vi "Remove Unused Connections.vi"(11 "TCP Slave in":refnum<class "TCP Server.lvclass">) -> (0 "error out":errorcluster)   [LabVIEW 2021, in "WebSockets.lvlib" / "TCP Server.lvclass"]
uses:
  TCP Server.lvclass
  TCP Server.lvclass/TCP Server.ctl
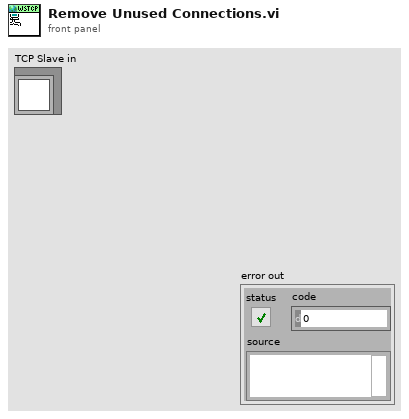
[diagram p1: front panel]
types:
  T1 = typedef "WebSockets.lvlib/TCP Server.lvclass/Connection Counter.ctl" = cluster{"Currently Connected":u32, "Connection Records":refnum<data-value>[]}
  T2 = typedef "WebSockets.lvlib/TCP Server.lvclass/Connection.ctl" = cluster{"Connected?":bool, "IP address":string, "connection error":errorcluster}
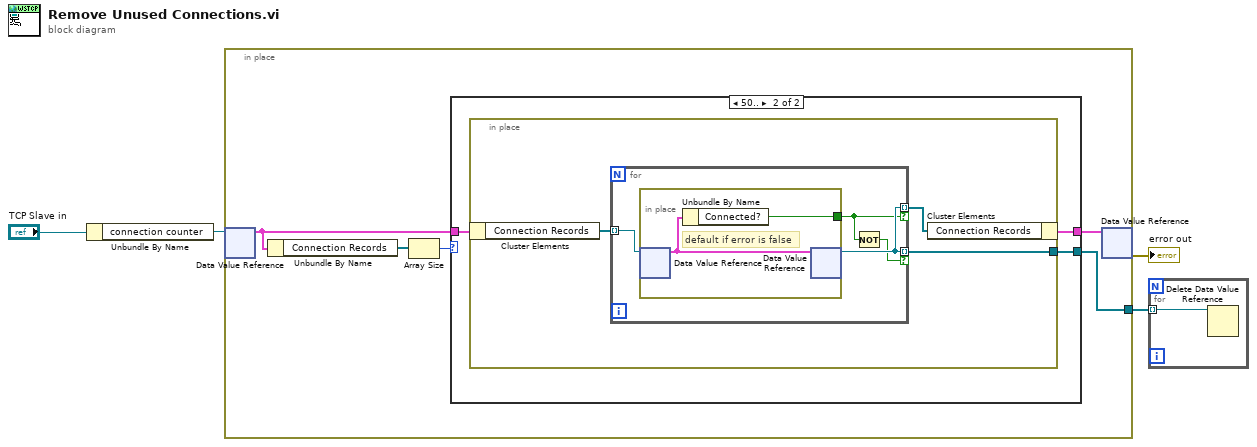
[diagram p0: block diagram]
diagram:
  n1 = Unbundle By Name("TCP Slave in") -> ("connection counter"=w2:refnum<data-value>)
  n2 = in-place {
    in-place-border: [w5] -> w1
    n3 = in-place-dvr #1(w2) -> (w6:T1)  [unwired: 1 out]
    n4 = Unbundle By Name(w6) -> ("Connection Records"=w8:refnum<data-value>[])
    n5 = Array Size(array=w8) -> (size(s)=w9:i32)
    n6 = case shown="50.." w9 {
      tunnel: [w10 w12] -> w7
      tunnel: w6 -> [w10 w13]
      tunnel: [_ w11] -> w5
      frame Default {
      }
      frame 50.. {
        n7 = in-place {
          in-place-border: [w14] -> w11
          n8 = in-place-cluster #2(w13) -> ("Connection Records"=w16:refnum<data-value>[])
          n9 = for {
            tunnel: w16 -> [w20] mode=indexing
            tunnel: [w19] -> w15 mode=indexing if=w18
            tunnel: [w19] -> w14 mode=indexing if=w17
            n10 = in-place {
              in-place-border: [w21] -> w18
              # "default if error is false"
              n11 = in-place-dvr #3(w20) -> (w22:T2)  [unwired: 1 out]
              n12 = Unbundle By Name(w22) -> ("Connected?"=w21:bool)
              n13 = in-place-dvr #3(w22) -> (w19:refnum<data-value>)  [unwired: 1 out]
            }
            n14 = Not(x=w18) -> (.not. x?=w17:bool)
          }
          n15 = in-place-cluster #2("Connection Records"=w15) -> (w12:T1)
        }
      }
    }
    n16 = in-place-dvr #1(w7) -> (→"error out":errorcluster)  [unwired: 1 out]
  }
  n17 = for {
    tunnel: w1 -> [w23] mode=indexing
    n18 = Delete Data Value Reference(data value reference=w23) -> ()  [unwired: 1 in, 2 out]
  }
